vi "ReadFiltHdrFiles_LS1.vi"(0 "nombre (-1)":i32=-1, 1 "Data Folder Path":path, 2 "ScanParamsIn":T1[](array[typedef]), 3 "VarParam":string, 5 "Date String":string="All" caption="Date String (yymmdd)", 9 "Session":i32=-1, 11 "error in (no error)":errorcluster, 12 "IncludeSubF":bool, 13 "Recheck Files":bool, 14 "KeyWord":string) -> (4 "ScanParamsOut":T1[](array[typedef]), 15 "error out":errorcluster)   [LabVIEW 2010]
doc: "Ce VI lit les données contenu dans le fichier de sauvegarde automatique. Ces données correspondent aux valeurs prises lors du dernier balayage. La sauvegarde automatique est effectué après chaque acquisition."
uses:
  Interface Class/ScanParams.ctl
  Interface Class/Interface.lvclass
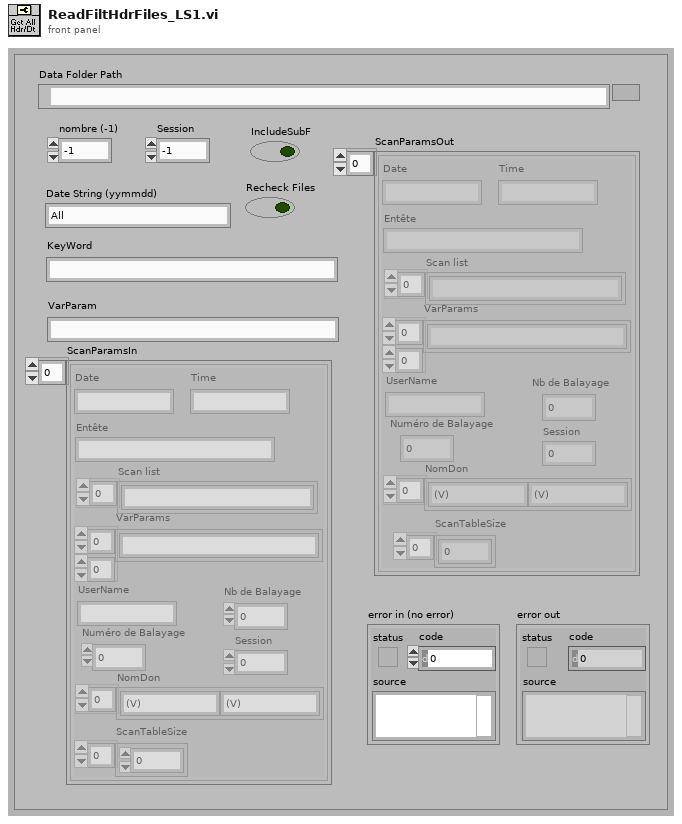
[diagram p1: front panel]
types:
  T1 = typedef "Interface.lvclass/ScanParams.ctl" = cluster{"Entête":string, "Scan list":string[], "NbCourbe":i32, "IndCourbe":i64, "NomDon":string[], "Session ":i32, "Date":string, "Time":string, "VarParams":string[][], "UserName":string, "ScanTableSize":i32[]}
  T2 = enum16{"open", "replace", "create", "open or create", "replace or create", "replace or create with confirmation"}
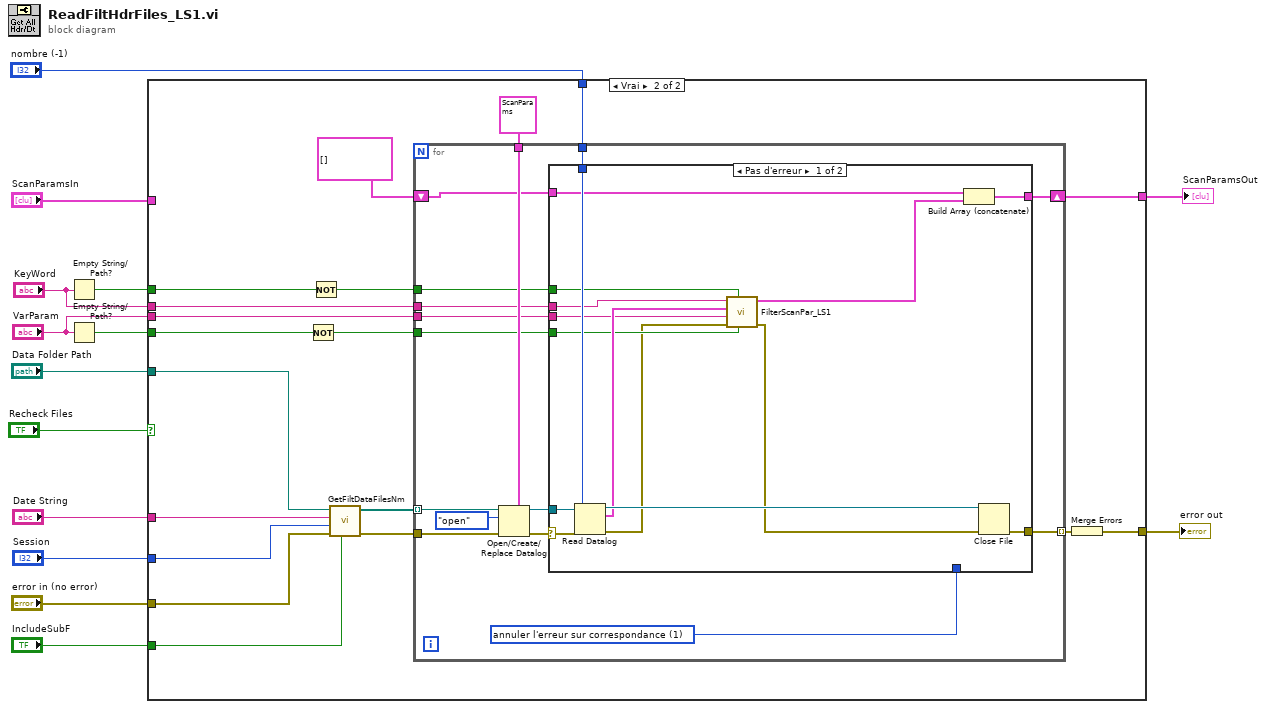
[diagram p0: block diagram]
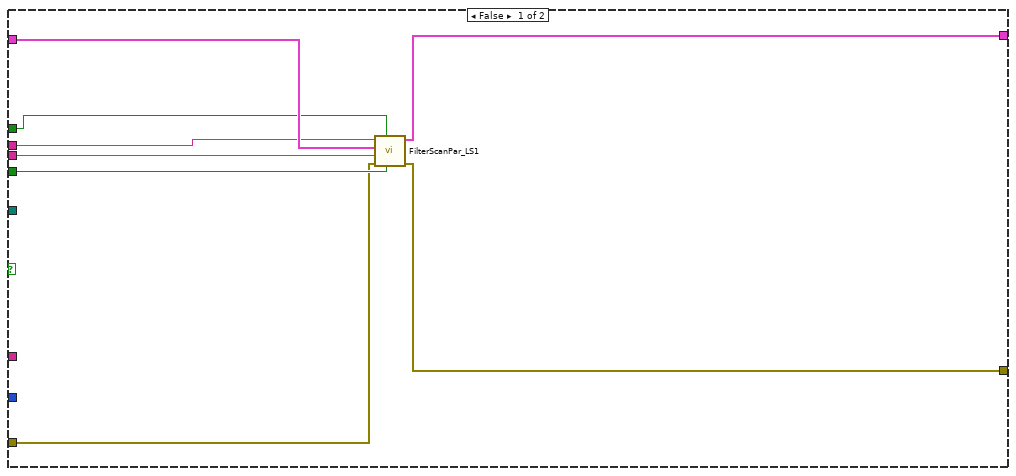
[diagram p2: hidden frame]
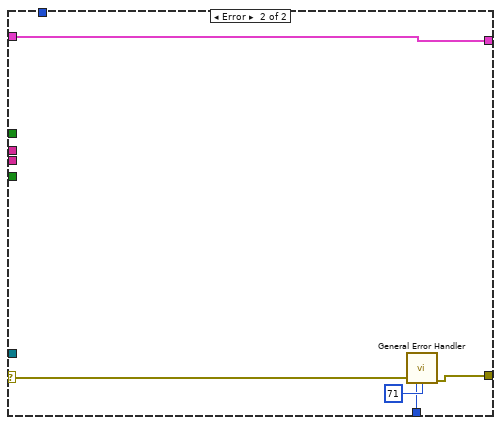
[diagram p3: hidden frame]
diagram:
  n1 = Empty String/Path?(string/path="KeyWord") -> (empty?=w6:bool)
  n2 = Empty String/Path?(string/path="VarParam") -> (empty?=w3:bool)
  n3 = case shown="Vrai" "Recheck Files" {
    tunnel: "nombre (-1)" -> [_ w40]
    tunnel: [w16 w38] -> w13
    tunnel: [w15 w36] -> w12
    tunnel: "Data Folder Path" -> [_ w35]
    tunnel: "Date String" -> [_ w34]
    tunnel: "error in (no error)" -> [w17 w33]
    tunnel: "Session" -> [_ w32]
    tunnel: "IncludeSubF" -> [_ w30]
    tunnel: w6 -> [w18 w28]
    tunnel: "KeyWord" -> [w19 w27]
    tunnel: "VarParam" -> [w20 w25]
    tunnel: w3 -> [w21 w24]
    tunnel: "ScanParamsIn" -> [w22 _]
    frame False {
      n4 = call "FilterScanPar_LS1.vi"("SearchVarPar"=w21, "SearchKey"=w18, "error in (no error)"=w17, "VarParam"=w20, "ScanParams"=w22, "KeyWord"=w19) -> ("error out"=w16:errorcluster, "ScanParamsOut"=w15:T1[])  [unwired: 4 in]
    }
    frame True {
      n5 = Not(x=w24) -> (.not. x?=w23:bool)
      n6 = Not(x=w28) -> (.not. x?=w26:bool)
      n7 = call "GetFiltDataFilesNm.vi"("IncludeSubF"=w30, "error in (no error)"=w33, "Session"=w32, "Date String"=w34, "Data Folder Path"=w35) -> ("error out"=w31:errorcluster, "HdrFilesNames"=w29:path[])  [unwired: 5 in]
      n8 = for {
        tunnel: [w56] -> w39 mode=indexing
        tunnel: T1 {"Entête"="", "Scan list"=[], "NbCourbe"=1, "IndCourbe"=1, "NomDon"=["RTêta;", "X&Y;"], "Session "=0, "Date"="", "Time"="", "VarParams"=[], "UserName"="", "ScanTableSize"=[]} ("ScanParams") -> [w55]
        tunnel: w40 -> [w52]
        tunnel: w31 -> [w47]
        shift-right: [w50] -> w36
        shift-left: T1[] [] -> [w51]
        tunnel: w29 -> [w46] mode=indexing
        tunnel: w26 -> [w45]
        tunnel: w27 -> [w44]
        tunnel: w25 -> [w43]
        tunnel: w23 -> [w42]
        w48 = 1 items=["pas d'exception", "annuler l'erreur sur correspondance", "définir l'erreur sur correspondance"] ("[exception action] (none:0)")
        n9 = Open/Create/Replace Datalog(5:w55, 8:w47, 10:T2."open" ("opération (0 : open)"), 11:w46) -> (0:w49:errorcluster, 3:w54:refnum<k1>)  [unwired: 2 in, 1 out]
        n10 = case shown="Pas d'erreur" w49 {
          selector: w49 -> [w66 w75]
          tunnel: [w71 w74] -> w56
          tunnel: w54 -> [w70 _]
          tunnel: w52 -> [w68 _]
          tunnel: w51 -> [w65 w76]
          tunnel: [w67 w76] -> w50
          tunnel: w48 -> [_ w72]
          tunnel: w45 -> [w61 _]
          tunnel: w44 -> [w60 _]
          tunnel: w43 -> [w63 _]
          tunnel: w42 -> [w62 _]
          frame No Error {
            n11 = Read Datalog(4:w66, 6:w68, 7:w70) -> (0:w59:errorcluster, 2:w64:T1[], 3:w69:refnum<k1>)
            n12 = call "FilterScanPar_LS1.vi"("SearchVarPar"=w62, "SearchKey"=w61, "error in (no error)"=w59, "VarParam"=w63, "ScanParams"=w64, "KeyWord"=w60) -> ("error out"=w58:errorcluster, "ScanParamsOut"=w57:T1[])  [unwired: 4 in]
            n13 = Build Array (concatenate)(w65, w57) -> (w67:T1[])
            n14 = Close File(refnum=w69, error in=w58) -> (error out=w71:errorcluster)  [unwired: 1 out]
          }
          frame Error {
            n15 = call <vilib>:"General Error Handler.vi"("error in (no error)"=w75, "[exception action] (none:0)"=w72, "[exception code]"=71) -> ("error out"=w74:errorcluster)  [unwired: 8 in, 4 out]
          }
        }
      }
      n16 = Merge Errors(w39) -> (w38:errorcluster)
    }
  }
  "error out" <- w13
  "ScanParamsOut" <- w12
